vi "Operation.vi"(8 "error in (no error)":errorcluster, 11 "ConcreteProductA in":refnum<class "ConcreteProductB.lvclass">) -> (0 "error out":errorcluster, 2 "ResultString":string, 3 "ConcreteProductA out":refnum<class "ConcreteProductB.lvclass">)   [LabVIEW 2020, in "FactoryMethod.lvlib" / "ConcreteProductB.lvclass"]
uses:
  ConcreteProductB.lvclass
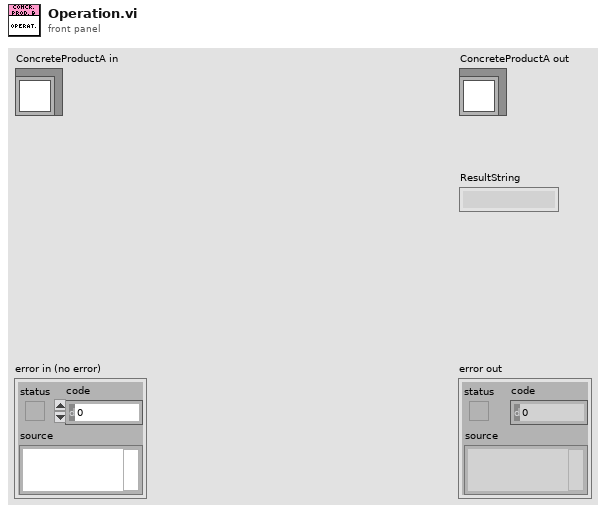
[diagram p1: front panel]
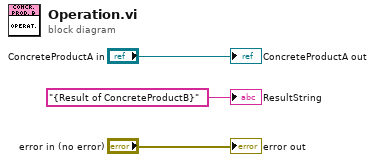
[diagram p0: block diagram]
diagram:
  "error out" <- "error in (no error)"
  "ConcreteProductA out" <- "ConcreteProductA in"
  "ResultString" <- "{Result of ConcreteProductB}" ("ResultString")
